vi "CSAFinishingConditionVi.vi"(0 "Specified \nTemperature\nLimit\nInput":dbl, 5 "Input Data":dbl[](array[numeric]), 7 "Time in s":dbl, 9 "prerun period":dbl) -> ()   [LabVIEW 2020]
panel:
  out "Dim 2":dbl[](array[numeric])
  out "30 min difference":dbl[](array[numeric])
  in  "Array 2":dbl[](array[numeric])
  out "Dim":dbl[](array[numeric])
  in  "Array":dbl[](array[numeric])
  out "5 min difference":dbl[](array[numeric])
  out "30 min ago":dbl[][](array[numeric])
  out "5 min ago":dbl[][](array[numeric])
  out "Unused":i32
  out "Row Count":i32
  out "Unused Data":dbl[](array[numeric])
  out "Incrementing \nIndicator":dbl
  out "current":dbl[][](array[numeric])
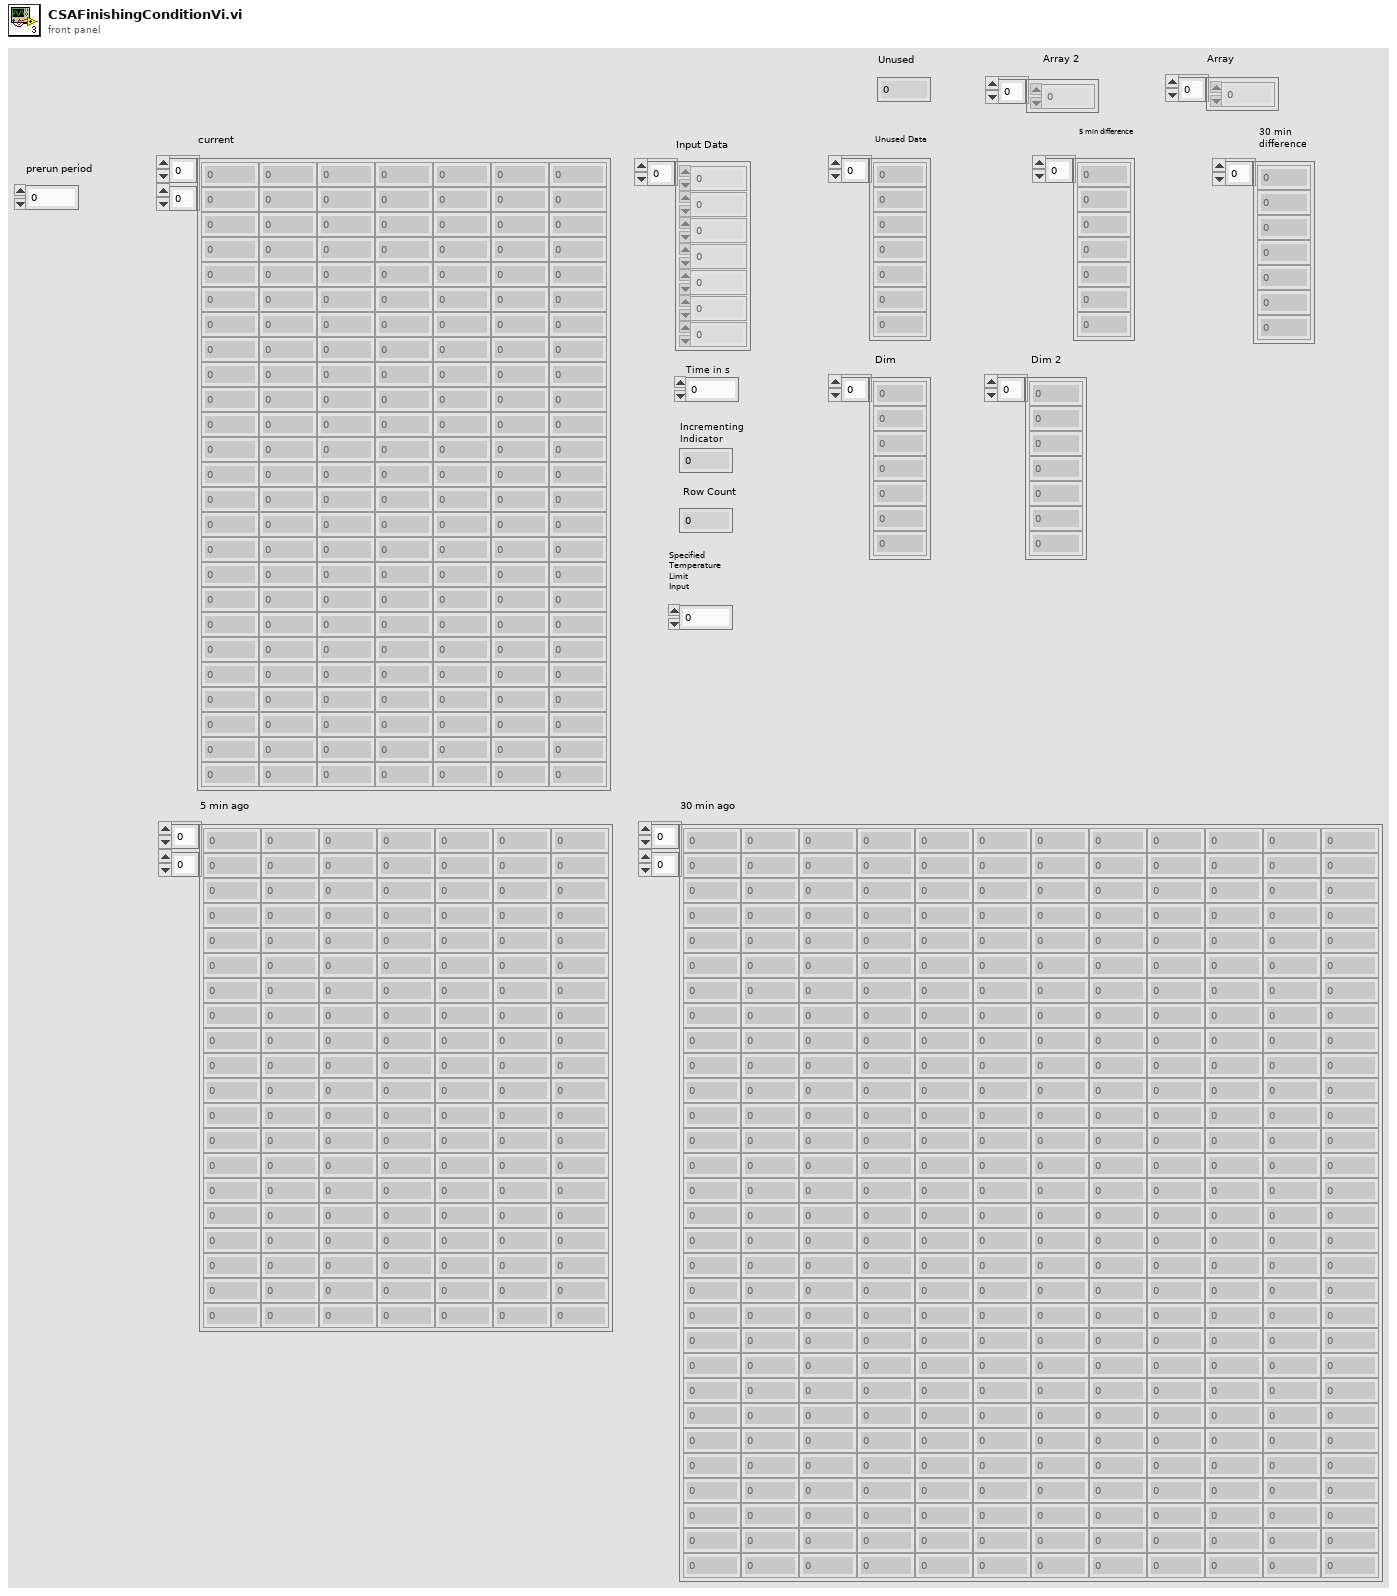
[diagram p1: front panel]
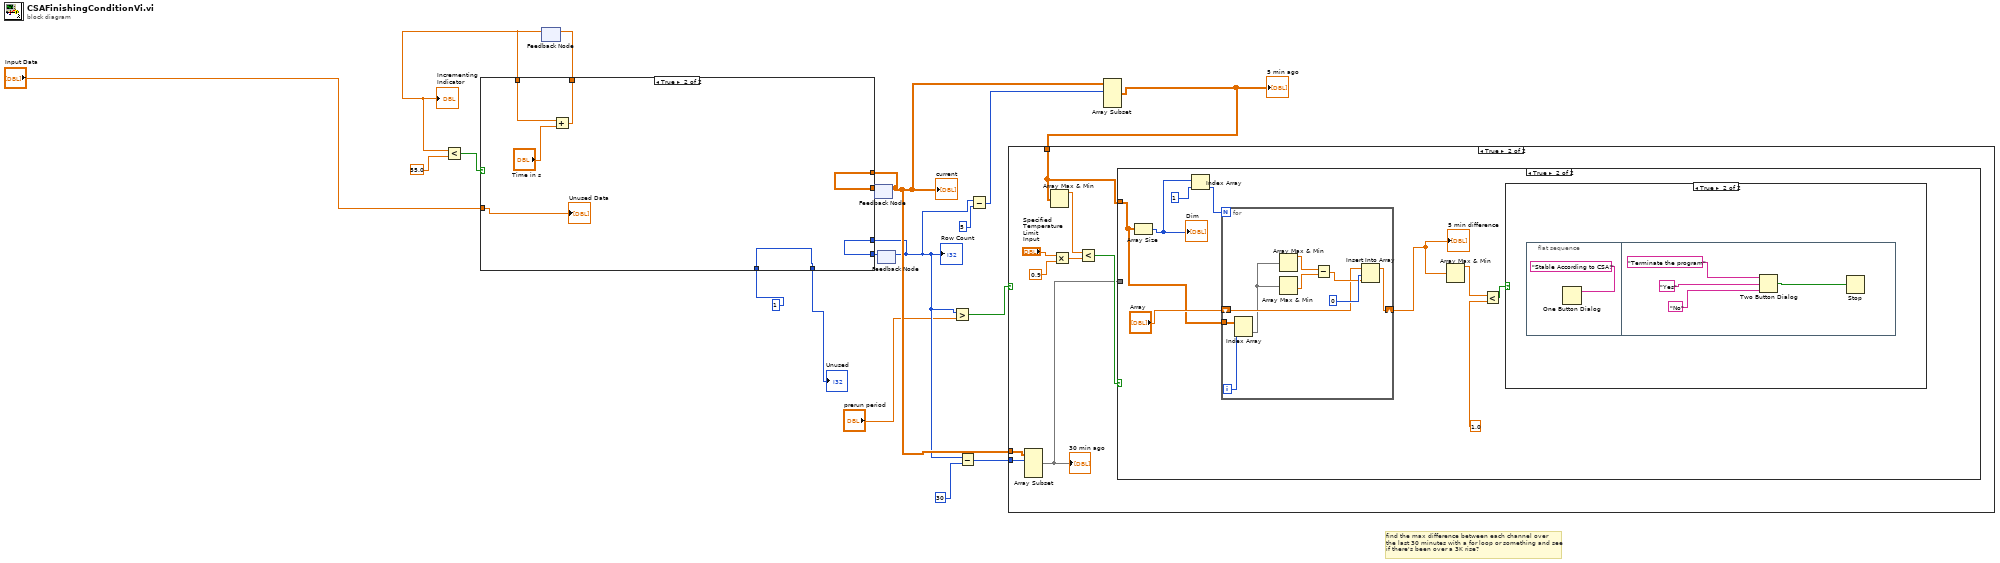
[diagram p0: block diagram]
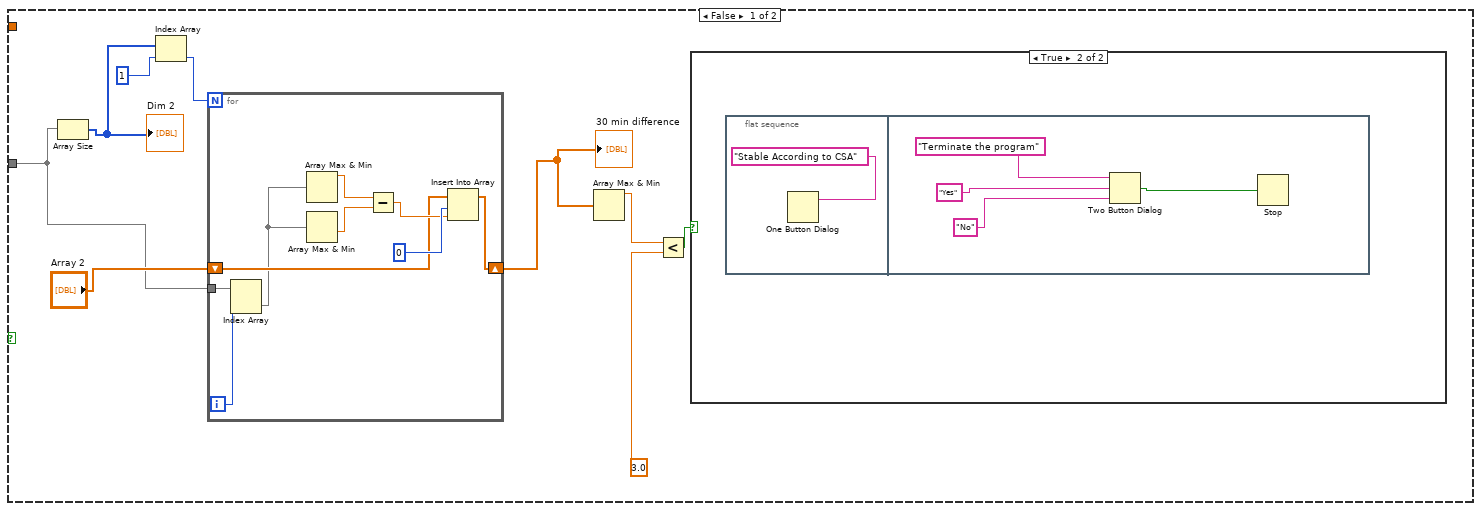
[diagram p3: hidden frame]
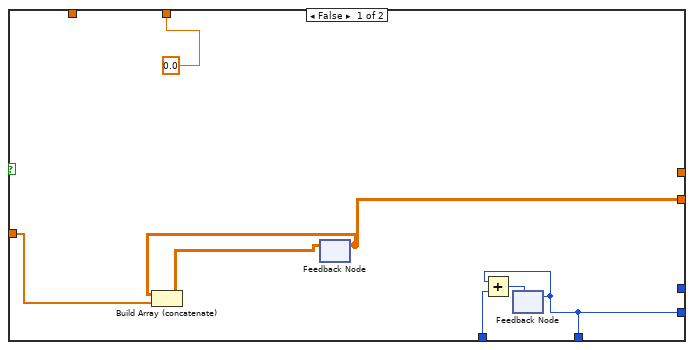
[diagram p6: hidden frame]
diagram:
  # "find the max difference between each channel over\nthe last 30 minutes with a for loop or something and see \nif there's been over a 3K rise?"
  n1 = feedback #1() -> (w10:dbl)  [unwired: 1 in]
  "Incrementing \nIndicator" <- w10
  n2 = Less?(x=w10, y=55.0) -> (x < y?=w17:bool)
  n3 = feedback #2() -> (w6:dbl[][])  [unwired: 1 in]
  "current" <- w6
  n4 = feedback #3() -> (w4:i32)  [unwired: 1 in]
  "Row Count" <- w4
  n5 = case shown="True" w17 {
    tunnel: "Input Data" -> [w25 w32]
    tunnel: 1 -> [w23 w29]
    tunnel: [w20 w29] -> w7
    tunnel: [w21 w31] -> w13
    tunnel: w6 -> [_ w31]
    tunnel: [w20 w30] -> w12
    tunnel: w4 -> [_ w30]
    tunnel: [0.0 w27] -> w11
    tunnel: w10 -> [_ w26]
    frame False {
      n6 = feedback #4() -> (w21:dbl[][])  [unwired: 1 in]
      n7 = Build Array (concatenate)(w21, w25) -> (w24:dbl[][])
      n8 = feedback-in #4(w24) -> ()
      n9 = feedback #5() -> (w20:i32)  [unwired: 1 in]
      n10 = Add(x=w20, y=w23) -> (x+y=w22:i32)
      n11 = feedback-in #5(w22) -> ()
    }
    frame True {
      n12 = Add(x=w26, y="Time in s") -> (x+y=w27:dbl)
      "Unused Data" <- w32
    }
  }
  "Unused" <- w7
  n13 = feedback-in #1(w11) -> ()
  n14 = feedback-in #2(w13) -> ()
  n15 = feedback-in #3(w12) -> ()
  n16 = Greater?(x=w4, y="prerun period") -> (0:w15:bool)
  n17 = Subtract(x=w4, y=30) -> (x-y=w8:i32)
  n18 = Subtract(x=w4, y=5) -> (x-y=w3:i32)
  n19 = Array Subset(array=w6, index (row)=w3) -> (w2:dbl[][])  [unwired: 3 in]
  "5 min ago" <- w2
  n20 = case shown="True" w15 {
    tunnel: w8 -> [_ w37]
    tunnel: w6 -> [_ w36]
    tunnel: w2 -> [_ w34]
    frame False {
    }
    frame True {
      n21 = Array Subset(array=w36, index (row)=w37) -> (w33:dbl[][])  [unwired: 3 in]
      "30 min ago" <- w33
      n22 = Array Max & Min(array=w34) -> (max value=w35:dbl)  [unwired: 3 out]
      n23 = Multiply(x="Specified \nTemperature\nLimit\nInput", y=0.9) -> (x*y=w41:dbl)
      n24 = Less?(x=w35, y=w41) -> (x < y?=w38:bool)
      n25 = case shown="True" w38 {
        tunnel: w34 -> [_ w65]
        tunnel: w33 -> [w42 _]
        frame False {
          n26 = Array Size(array=w42) -> (size(s)=w45:i32[])
          "Dim 2" <- w45
          n27 = Index Array(array=w45, index=1) -> (element=w43:i32)
          n28 = for {
            N: w43 -> [_]
            shift-right: [w54] -> w47
            shift-left: "Array 2" -> [w55]
            tunnel: w42 -> [w52]
            i -> [w53]
            n29 = Index Array(array=w52, index (col)=w53) -> (element=w51:dbl[])  [unwired: 1 in]
            n30 = Array Max & Min(array=w51) -> (max value=w59:dbl)  [unwired: 3 out]
            n31 = Array Max & Min(array=w51) -> (min value=w58:dbl)  [unwired: 3 out]
            n32 = Subtract(x=w59, y=w58) -> (x-y=w56:dbl)
            n33 = Insert Into Array(array=w55, index=0, new element=w56) -> (w54:dbl[])
          }
          "30 min difference" <- w47
          n34 = Array Max & Min(array=w47) -> (max value=w46:dbl)  [unwired: 3 out]
          n35 = Less?(x=w46, y=3.0) -> (x < y?=w49:bool)
          n36 = case shown="True" w49 {
            frame False {
            }
            frame True {
              n37 = flat-sequence {
                frame #0 {
                  n38 = One Button Dialog(message="Stable According to CSA") -> ()  [unwired: 1 in, 1 out]
                }
                frame #1 {
                  n39 = Two Button Dialog(message="Terminate the program", 1:"No", 2:"Yes") -> (T button?=w61:bool)
                  n40 = Stop(stop? (T)=w61) -> ()
                }
              }
            }
          }
        }
        frame True {
          n41 = Array Size(array=w65) -> (size(s)=w68:i32[])
          "Dim" <- w68
          n42 = Index Array(array=w68, index=1) -> (element=w66:i32)
          n43 = for {
            N: w66 -> [_]
            shift-right: [w77] -> w70
            shift-left: "Array" -> [w78]
            tunnel: w65 -> [w75]
            i -> [w76]
            n44 = Index Array(array=w75, index (col)=w76) -> (element=w74:dbl[])  [unwired: 1 in]
            n45 = Array Max & Min(array=w74) -> (max value=w82:dbl)  [unwired: 3 out]
            n46 = Array Max & Min(array=w74) -> (min value=w81:dbl)  [unwired: 3 out]
            n47 = Subtract(x=w82, y=w81) -> (x-y=w79:dbl)
            n48 = Insert Into Array(array=w78, index=0, new element=w79) -> (w77:dbl[])
          }
          "5 min difference" <- w70
          n49 = Array Max & Min(array=w70) -> (max value=w69:dbl)  [unwired: 3 out]
          n50 = Less?(x=w69, y=1.0) -> (x < y?=w72:bool)
          n51 = case shown="True" w72 {
            frame False {
            }
            frame True {
              n52 = flat-sequence {
                frame #0 {
                  n53 = One Button Dialog(message="Stable According to CSA!") -> ()  [unwired: 1 in, 1 out]
                }
                frame #1 {
                  n54 = Two Button Dialog(message="Terminate the program", 1:"No", 2:"Yes") -> (T button?=w84:bool)
                  n55 = Stop(stop? (T)=w84) -> ()
                }
              }
            }
          }
        }
      }
    }
  }
